vi "Compare within Relative Epsilon.vi"(9 "Rel Epsilon":dbl, 10 "b":dbl, 11 "a":dbl) -> (2 "|a – b|/|b|":dbl, 3 "a == b?":bool)   [LabVIEW 2014, in "Endigit.lvlib"]
uses:
  Endigit.lvlib
panel:
  # "NOTICE - YOU MUST NOT REMOVE THIS NOTICE. PER THE FOLLOWING LICENSE, YOU MAY REPRODUCE THIS SOFTWARE PROVIDED YOU FOLLOW THE TERMS\nOF THE LICENSE.\n\n---BEGIN BSD LICENSE (http://opensource.org/licenses/BSD-2-Clause)---\nCopyright (c) 2015, Endigit, Inc. <robert@endigit.com>\nAll rights reserved.\n\nRedistribution and use in source and binary forms, with or without modification, are permitted provided that the following conditions are met:\n\n1. Redistributions of source code must retain the above copyright notice, this list of conditions and the following disclaimer.\n\n2. Redistributions in binary form must reproduce the above copyright notice, this list of conditions and the following disclaimer in the documentation and/or other \nmaterials provided with the distribution.\n\nTHIS SOFTWARE IS PROVIDED BY THE COPYRIGHT HOLDERS AND CONTRIBUTORS \"AS IS\" AND ANY EXPRESS OR IMPLIED WARRANTIES, INCLUDING, BUT NOT \nLIMITED TO, THE IMPLIED WARRANTIES OF MERCHANTABILITY AND FITNESS FOR A PARTICULAR PURPOSE ARE DISCLAIMED. IN NO EVENT SHALL THE COPYRIGHT \nHOLDER OR CONTRIBUTORS BE LIABLE FOR ANY DIRECT, INDIRECT, INCIDENTAL, SPECIAL, EXEMPLARY, OR CONSEQUENTIAL DAMAGES (INCLUDING, BUT NOT \nLIMITED TO, PROCUREMENT OF SUBSTITUTE GOODS OR SERVICES; LOSS OF USE, DATA, OR PROFITS; OR BUSINESS INTERRUPTION) HOWEVER CAUSED AND ON \nANY THEORY OF LIABILITY, WHETHER IN CONTRACT, STRICT LIABILITY, OR TORT (INCLUDING NEGLIGENCE OR OTHERWISE) ARISING IN ANY WAY OUT OF THE USE \nOF THIS SOFTWARE, EVEN IF ADVISED OF THE POSSIBILITY OF SUCH DAMAGE.\n---END BSD LICENSE---"
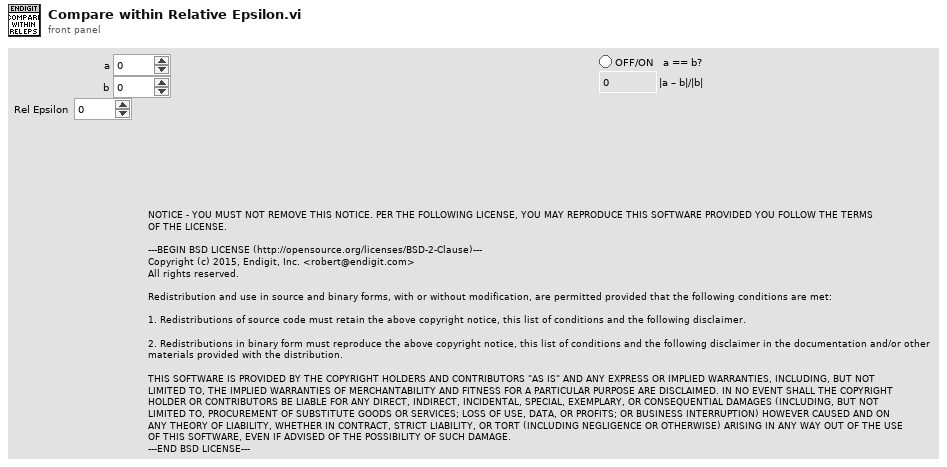
[diagram p1: front panel]
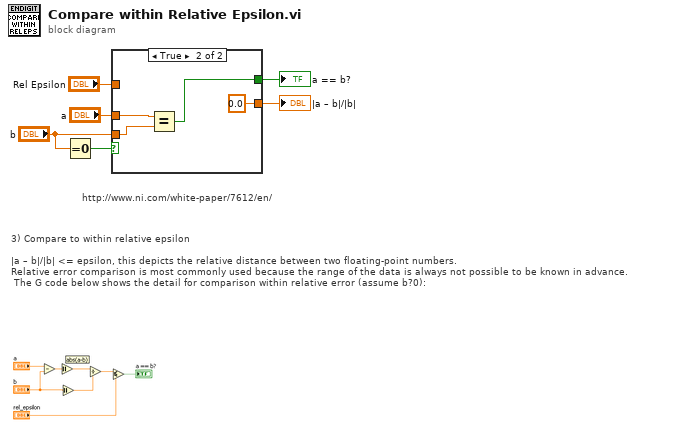
[diagram p0: block diagram]
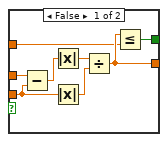
[diagram p2: hidden frame]
diagram:
  # "http://www.ni.com/white-paper/7612/en/"
  # "3) Compare to within relative epsilon\n\n|a – b|/|b| <= epsilon, this depicts the relative distance between two floating-point numbers. \nRelative error comparison is most commonly used because the range of the data is always not possible to be known in advance.\n The G code below shows the detail for comparison within relative error (assume b?0):"
  n1 = Equal To 0?(x="b") -> (x = 0?=w1:bool)
  n2 = case shown="True" w1 {
    tunnel: "a" -> [w14 w18]
    tunnel: [w10 0.0] -> w5
    tunnel: "Rel Epsilon" -> [w9 _]
    tunnel: [w8 w16] -> w3
    tunnel: "b" -> [w7 w17]
    frame False {
      n3 = Subtract(x=w14, y=w7) -> (x-y=w13:dbl)
      n4 = Absolute Value(x=w13) -> (abs(x)=w12:dbl)
      n5 = Absolute Value(x=w7) -> (abs(x)=w11:dbl)
      n6 = Divide(x=w12, y=w11) -> (x/y=w10:dbl)
      n7 = Less Or Equal?(x=w10, y=w9) -> (x <= y?=w8:bool)
    }
    frame True {
      n8 = Equal?(x=w18, y=w17) -> (x = y?=w16:bool)
    }
  }
  "a == b?" <- w3
  "|a – b|/|b|" <- w5
